vi "Inlet Valve Select Sub.vi"(9 "Valve control":bool, 10 "Valve select":T1, 11 "FPGA ref in":refnum<k20>) -> (3 "FPGA VI Reference Out":refnum<k20>)   [LabVIEW 2013]
uses:
  Types Def/Sample Inlet Valve.ctl
  <vilib>/rvi/interface/common/niFpgaWaitOnOcc.vi
  <vilib>/Utility/error.llb/Error Cluster From Error Code.vi
  <vilib>/rvi/errors/niLvFpgaAdjustHostInterfaceError.vi
  <vilib>/rvi/interface/nirviReadWriteControl/nirviReadWriteControl.xnode
  NiFpgaLv.dll
  <vilib>/rvi/interface/Simulation/niFpgaSimulationCallBeginRW.vi
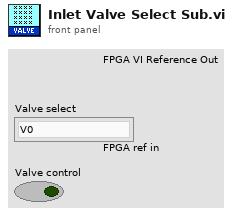
[diagram p1: front panel]
types:
  T1 = typedef "Sample Inlet Valve.ctl" = enum16{"V0", "V1", "V2", "V3", "V4", "V5", "V6", "V7", "V8", "V9", "V10", "V11", "V12", "V13", "V14", "V15", "VSTD1", "VSTD2", "VA"}
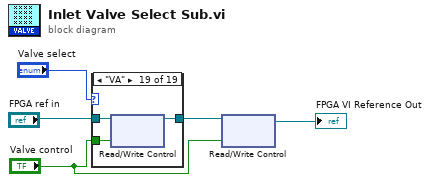
[diagram p0: block diagram]
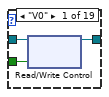
[diagram p2: hidden frame]
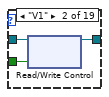
[diagram p3: hidden frame]
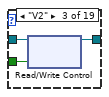
[diagram p4: hidden frame]
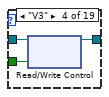
[diagram p5: hidden frame]
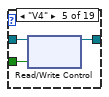
[diagram p6: hidden frame]
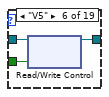
[diagram p7: hidden frame]
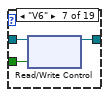
[diagram p8: hidden frame]
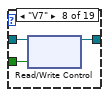
[diagram p9: hidden frame]
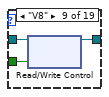
[diagram p10: hidden frame]
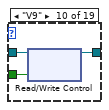
[diagram p11: hidden frame]
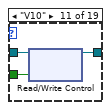
[diagram p12: hidden frame]
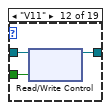
[diagram p13: hidden frame]
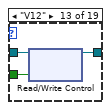
[diagram p14: hidden frame]
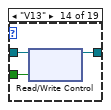
[diagram p15: hidden frame]
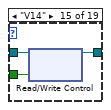
[diagram p16: hidden frame]
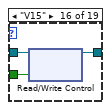
[diagram p17: hidden frame]
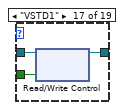
[diagram p18: hidden frame]
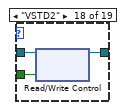
[diagram p19: hidden frame]
diagram:
  n1 = case shown="\"VA\"" "Valve select" {
    tunnel: "FPGA ref in" -> [w8 w11 w14 w17 w20 w23 w26 w29 w32 w35 w38 w41 w44 w47 w50 w53 w56 w59 w62]
    tunnel: "Valve control" -> [w6 w9 w12 w15 w18 w21 w24 w27 w30 w33 w36 w39 w42 w45 w48 w51 w54 w57 w60]
    tunnel: [w7 w10 w13 w16 w19 w22 w25 w28 w31 w34 w37 w40 w43 w46 w49 w52 w55 w58 w61] -> w4
    frame "V0" {
      n2 = xnode "Read/Write Control"("FPGA VI Reference In"=w8, "V0"=w6) -> ("FPGA VI Reference Out"=w7:refnum<k20>)  [unwired: 1 in, 1 out]
    }
    frame "V1" {
      n3 = xnode "Read/Write Control"("FPGA VI Reference In"=w11, "V1"=w9) -> ("FPGA VI Reference Out"=w10:refnum<k20>)  [unwired: 1 in, 1 out]
    }
    frame "V2" {
      n4 = xnode "Read/Write Control"("FPGA VI Reference In"=w14, "V2"=w12) -> ("FPGA VI Reference Out"=w13:refnum<k20>)  [unwired: 1 in, 1 out]
    }
    frame "V3" {
      n5 = xnode "Read/Write Control"("FPGA VI Reference In"=w17, "V3"=w15) -> ("FPGA VI Reference Out"=w16:refnum<k20>)  [unwired: 1 in, 1 out]
    }
    frame "V4" {
      n6 = xnode "Read/Write Control"("FPGA VI Reference In"=w20, "V4"=w18) -> ("FPGA VI Reference Out"=w19:refnum<k20>)  [unwired: 1 in, 1 out]
    }
    frame "V5" {
      n7 = xnode "Read/Write Control"("FPGA VI Reference In"=w23, "V5"=w21) -> ("FPGA VI Reference Out"=w22:refnum<k20>)  [unwired: 1 in, 1 out]
    }
    frame "V6" {
      n8 = xnode "Read/Write Control"("FPGA VI Reference In"=w26, "V6"=w24) -> ("FPGA VI Reference Out"=w25:refnum<k20>)  [unwired: 1 in, 1 out]
    }
    frame "V7" {
      n9 = xnode "Read/Write Control"("FPGA VI Reference In"=w29, "V7"=w27) -> ("FPGA VI Reference Out"=w28:refnum<k20>)  [unwired: 1 in, 1 out]
    }
    frame "V8" {
      n10 = xnode "Read/Write Control"("FPGA VI Reference In"=w32, "V8"=w30) -> ("FPGA VI Reference Out"=w31:refnum<k20>)  [unwired: 1 in, 1 out]
    }
    frame "V9" {
      n11 = xnode "Read/Write Control"("FPGA VI Reference In"=w35, "V9"=w33) -> ("FPGA VI Reference Out"=w34:refnum<k20>)  [unwired: 1 in, 1 out]
    }
    frame "V10" {
      n12 = xnode "Read/Write Control"("FPGA VI Reference In"=w38, "V10"=w36) -> ("FPGA VI Reference Out"=w37:refnum<k20>)  [unwired: 1 in, 1 out]
    }
    frame "V11" {
      n13 = xnode "Read/Write Control"("FPGA VI Reference In"=w41, "V11"=w39) -> ("FPGA VI Reference Out"=w40:refnum<k20>)  [unwired: 1 in, 1 out]
    }
    frame "V12" {
      n14 = xnode "Read/Write Control"("FPGA VI Reference In"=w44, "V12"=w42) -> ("FPGA VI Reference Out"=w43:refnum<k20>)  [unwired: 1 in, 1 out]
    }
    frame "V13" {
      n15 = xnode "Read/Write Control"("FPGA VI Reference In"=w47, "V13"=w45) -> ("FPGA VI Reference Out"=w46:refnum<k20>)  [unwired: 1 in, 1 out]
    }
    frame "V14" {
      n16 = xnode "Read/Write Control"("FPGA VI Reference In"=w50, "V14"=w48) -> ("FPGA VI Reference Out"=w49:refnum<k20>)  [unwired: 1 in, 1 out]
    }
    frame "V15" {
      n17 = xnode "Read/Write Control"("FPGA VI Reference In"=w53, "V15"=w51) -> ("FPGA VI Reference Out"=w52:refnum<k20>)  [unwired: 1 in, 1 out]
    }
    frame "VSTD1" {
      n18 = xnode "Read/Write Control"("FPGA VI Reference In"=w56, "VSTD1"=w54) -> ("FPGA VI Reference Out"=w55:refnum<k20>)  [unwired: 1 in, 1 out]
    }
    frame "VSTD2" {
      n19 = xnode "Read/Write Control"("FPGA VI Reference In"=w59, "VSTD2"=w57) -> ("FPGA VI Reference Out"=w58:refnum<k20>)  [unwired: 1 in, 1 out]
    }
    frame "VA" {
      n20 = xnode "Read/Write Control"("FPGA VI Reference In"=w62, "VA"=w60) -> ("FPGA VI Reference Out"=w61:refnum<k20>)  [unwired: 1 in, 1 out]
    }
  }
  n21 = xnode "Read/Write Control"("FPGA VI Reference In"=w4, "VGPU"="Valve control") -> ("FPGA VI Reference Out"=→"FPGA VI Reference Out":refnum<k20>)  [unwired: 1 in, 1 out]
